vi "phy_dsss_chips.vi"(11 "symbols":cdb[](array[numeric])) -> (3 "chips":cdb[](array[numeric]))   [LabVIEW 2014]
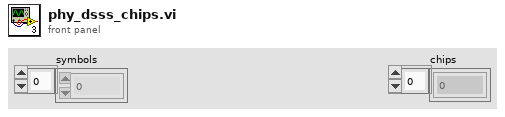
[diagram p1: front panel]
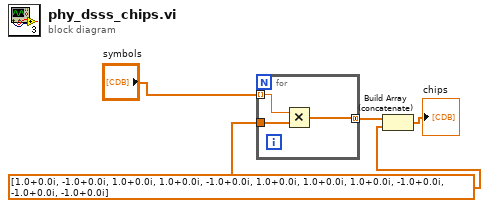
[diagram p0: block diagram]
diagram:
  w2 = cdb[] [1.0+0.0i, -1.0+0.0i, 1.0+0.0i, 1.0+0.0i, -1.0+0.0i, 1.0+0.0i, 1.0+0.0i, 1.0+0.0i, -1.0+0.0i, -1.0+0.0i, -1.0+0.0i]
  n1 = for {
    tunnel: "symbols" -> [w6] mode=indexing
    tunnel: w2 -> [w7]
    tunnel: [w5] -> w3 mode=concatenating
    n2 = Multiply(x=w6, y=w7) -> (x*y=w5:cdb[])
  }
  n3 = Build Array (concatenate)(w3, w2) -> (→"chips":cdb[])
